vi "SRV_PM_Get Data Field Length.vi"(0 "Packet":u8[](array[numeric]) format="%.0x", 11 "error in (no error)":errorcluster) -> (4 "Packet Data dup":u8[](array[numeric]) format="%.0x", 6 "Data Field Length":u16 format="%.0x", 15 "error out":errorcluster)   [LabVIEW 2009]
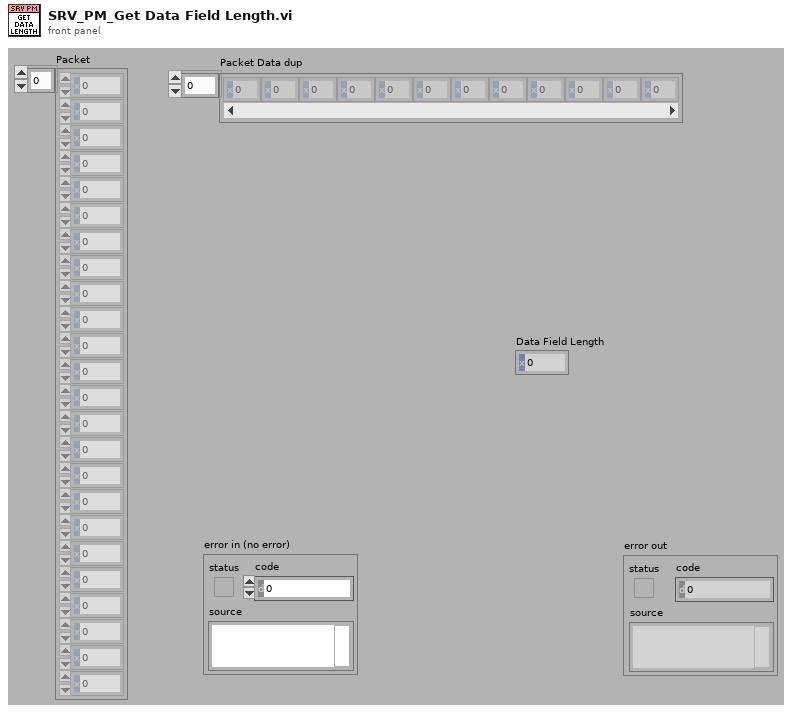
[diagram p1: front panel]
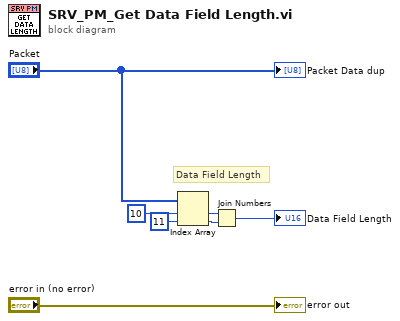
[diagram p0: block diagram]
diagram:
  # "Data Field Length"
  n1 = Index Array(array="Packet", index #1=10 ("index"), index #2=11 ("index")) -> (element #1=w6:u8, element #2=w5:u8)
  n2 = Join Numbers(hi=w6, lo=w5) -> ((hi.lo)=→"Data Field Length":u16)
  "error out" <- "error in (no error)"
  "Packet Data dup" <- "Packet"
